vi "Final_LabView.vi"() -> ()   [LabVIEW 2020]
uses:
  <vilib>/Utility/file.llb/Write Delimited Spreadsheet (DBL).vi
panel:
  in  "B_min":dbl=380.0
  in  "B_max":dbl=1420.0
  in  "G_min":dbl=365.0
  in  "G_max":dbl=1500.0
  in  "R_min":dbl=280.0
  in  "R_max":dbl=1450.0
  out "B_RAW":string="00386"
  out "G_RAW":string="00443"
  out "R_RAW":string="01267"
  out "data out":string="\r\n"
  out "B":dbl=253.52884615384616
  out "G":dbl=237.47577092511014
  out "R":dbl=39.88461538461539
  out "Color":u32(colorbox)=2682366
  in  "stop":bool
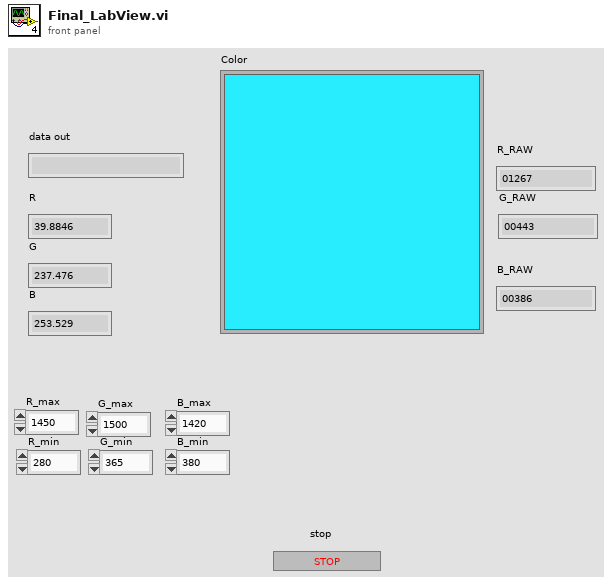
[diagram p1: front panel]
types:
  T1 = enum16{"Standard", "Buffered", "CRLF", "Immediate"}
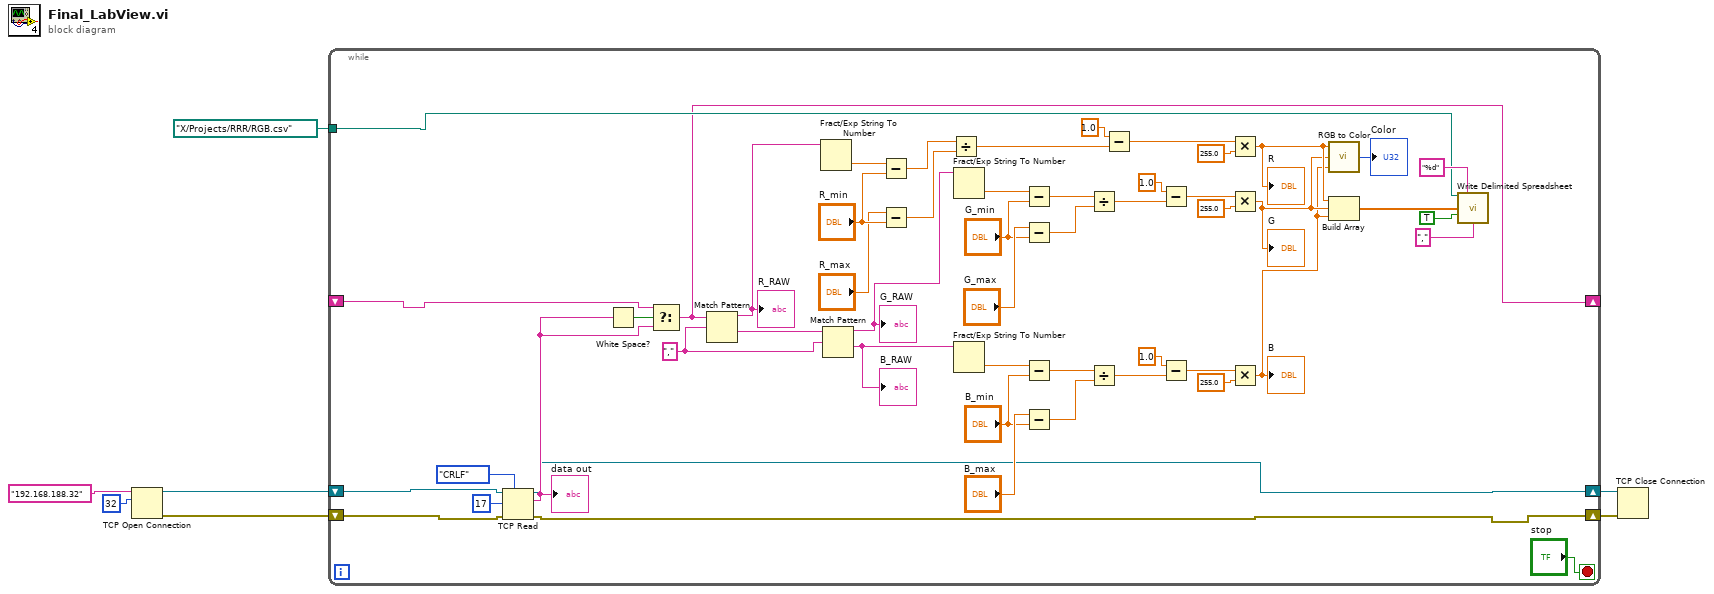
[diagram p0: block diagram]
diagram:
  n1 = TCP Open Connection(address="192.168.188.32", remote port or service name=u16 32) -> (connection ID=w7:refnum<k5>, error out=w6:errorcluster)  [unwired: 3 in]
  n2 = while {
    tunnel: path "X:/Projects/RRR/RGB.csv" ("file path (dialog if empty)") -> [w15]
    shift-right: [w12] -> w2
    shift-left: w7 -> [w9]
    shift-right: [w11] -> w1
    shift-left: w6 -> [w10]
    shift-right: [w13] -> _
    shift-left: _ -> [w14]
    stop <- "stop" stop-if-true
    w35 = "," ("regular expression")
    n3 = TCP Read(connection ID=w9, bytes to read=17, error in (no error)=w10, 7:T1."CRLF" ("mode (standard)")) -> (connection ID out=w12:refnum<k5>, data out=w28:string, error out=w11:errorcluster)  [unwired: 1 in]
    "data out" <- w28
    n4 = White Space?(1:w28) -> (0:w29:bool)
    n5 = Select(t=w14, s=w29, f=w28) -> (s? t:f=w13:string)
    n6 = Match Pattern(string=w13, regular expression=w35) -> (before substring=w38:string, after substring=w36:string)  [unwired: 1 in, 2 out]
    "R_RAW" <- w38
    n7 = Fract/Exp String To Number(string=w38) -> (number=w33:dbl)  [unwired: 3 in, 1 out]
    n8 = Match Pattern(string=w36, regular expression=w35) -> (before substring=w37:string, after substring=w34:string)  [unwired: 1 in, 2 out]
    "G_RAW" <- w37
    "B_RAW" <- w34
    n9 = Subtract(x=w33, y="R_min") -> (x-y=w58:dbl)
    n10 = Subtract(x="R_max", y="R_min") -> (x-y=w52:dbl)
    n11 = Divide(x=w58, y=w52) -> (x/y=w27:dbl)
    n12 = Fract/Exp String To Number(string=w37) -> (number=w32:dbl)  [unwired: 3 in, 1 out]
    n13 = Fract/Exp String To Number(string=w34) -> (number=w31:dbl)  [unwired: 3 in, 1 out]
    n14 = Subtract(x=w32, y="G_min") -> (x-y=w49:dbl)
    n15 = Subtract(x="G_max", y="G_min") -> (x-y=w48:dbl)
    n16 = Subtract(x=w31, y="B_min") -> (x-y=w57:dbl)
    n17 = Subtract(x="B_max", y="B_min") -> (x-y=w45:dbl)
    n18 = Divide(x=w49, y=w48) -> (x/y=w22:dbl)
    n19 = Divide(x=w57, y=w45) -> (x/y=w20:dbl)
    n20 = Subtract(x=1.0, y=w27) -> (x-y=w25:dbl)
    n21 = Subtract(x=1.0, y=w22) -> (x-y=w21:dbl)
    n22 = Subtract(x=1.0, y=w20) -> (x-y=w19:dbl)
    n23 = Multiply(x=w25, y=255.0) -> (x*y=w43:dbl)
    "R" <- w43
    n24 = Multiply(x=w21, y=255.0) -> (x*y=w42:dbl)
    "G" <- w42
    n25 = Multiply(x=w19, y=255.0) -> (x*y=w41:dbl)
    "B" <- w41
    n26 = call <vilib>:"RGB to Color.vi"("B"=w41, "G"=w42, "R"=w43) -> ("Color"=→"Color":u32)
    n27 = Build Array "Build Array"(w43, w42, w41) -> (w16:dbl[])
    n28 = call-poly <vilib>:"Write Delimited Spreadsheet.vi"("file path (dialog if empty)"=w15, "format (%.3f)"="%d", "1D data"=w16, "append to file? (new file:F)"=TRUE, "delimiter (\\t)"="," ("delimiter (\\t)")) -> ()  [unwired: 9 in, 2 out]
  }
  n29 = TCP Close Connection(connection ID=w2, error in (no error)=w1) -> ()  [unwired: 1 in, 2 out]
